vi "cRIO Example FPGA.vi"() -> ()   [LabVIEW 2024]
uses:
  <vilib>/Platform/TimedLoop/XDataNode/timing_clust.ctl
  <vilib>/Platform/TimedLoop/XDataNode/nitl_modes.ctl
  <vilib>/Platform/TimedLoop/XDataNode/wakeup.ctl
  <vilib>/rvi/Emulation/niFpgaSctlEmulationGetInTimedLoop.vi
  <vilib>/rvi/Emulation/niFpgaEmulationReportErrorSimple.vi
  <vilib>/rvi/Emulation/niFpgaGetClockAttributes.vi
  <vilib>/rvi/Emulation/niFpgaCriticalErrorInLSC.vi
  <vilib>/rvi/Emulation/niFpgaProcessEmulError.vi
  <vilib>/rvi/eio/common/nirviEmuTemplateMethod_errors.vi
  <userlib>/_VeriStand FPGA XML Builder/Boolean Array to U64.vi
  <vilib>/NI VeriStand/FPGA/NI VeriStand - Send Packet to Host.vi
  <vilib>/Platform/TimedLoop/XDataNode/XDataNode.xnode
  <vilib>/eio/EIONode/EIONode.xnode
  <userlib>/_VeriStand FPGA XML Builder/FPGA XML.xnode
  <vilib>/Platform/TimedLoop/XDataNode/XDNodeRunTimeDep.lvlib
  <vilib>/NI VeriStand/FPGA/NI_VS FPGA Support.lvlib
panel:
  in  "PulseMeas 0 Timeout":u32=40000
  out "PulseMeas Packet":u64
  in  "Loop Rate (ticks)":u32
  in  "Start":bool
  # "PWM"
  # "Configuration"
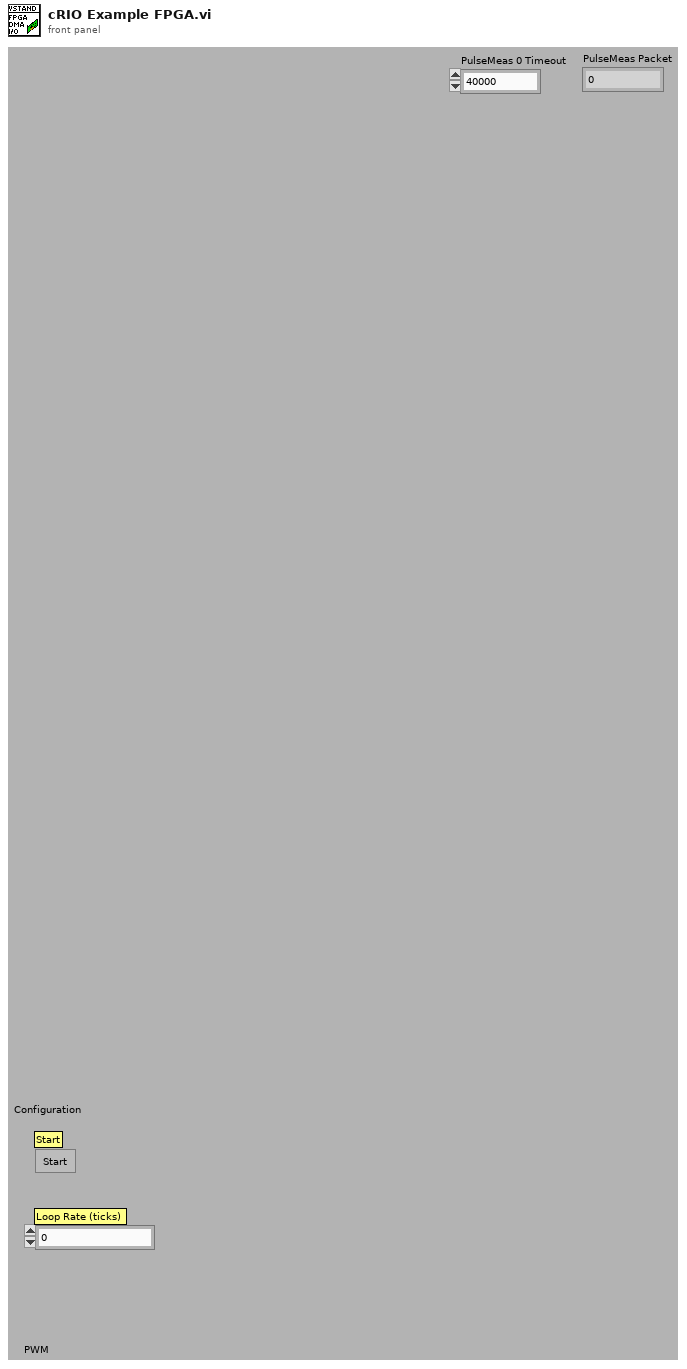
[diagram p1: front panel]
types:
  T1 = typedef "XDNodeRunTimeDep.lvlib/timing_clust.ctl" = cluster{"Expected End [f-1]":u64, "Actual End [f-1]":u64, "Finished Late? [f-1]":bool, "Expected End [i-1]":u64, "Actual End [i-1]":u64, "Finished Late? [i-1]":bool, "Expected Start [i]":u64, "Actual Start [i]":u64, "Expected Start [f]":u64, "Actual Start [f]":u64, "Source Name":string, "Structure Name":string, "Period":i64, "Deadline":i64, "Offset":i64, "Start":i64, "Priority":i32, "Timeout":i32, "Mode":T2, "Wakeup Reason":T3, "Error":errorcluster, "Source Type":string, "Secondary Source Type":string, "Global End Time":u64, "Global Start Time":u64, "Frame Duration":u64, "Iteration Duration":u64, "Assigned CPU":i32, "I/O Scan Engine Mode":u32}
  T2 = typedef "XDNodeRunTimeDep.lvlib/nitl_modes.ctl" = enum32{"No Change", "Process missed periods, maintain original phase", "Discard missed periods, maintain original phase", "Process missed periods, ignore original phase", "Discard missed periods, ignore original phase"}
  T3 = typedef "XDNodeRunTimeDep.lvlib/wakeup.ctl" = enum32{"Normal", "Aborted", "Asynchronous wakeup", "Timing source error", "Timed loop error", "Timeout"}
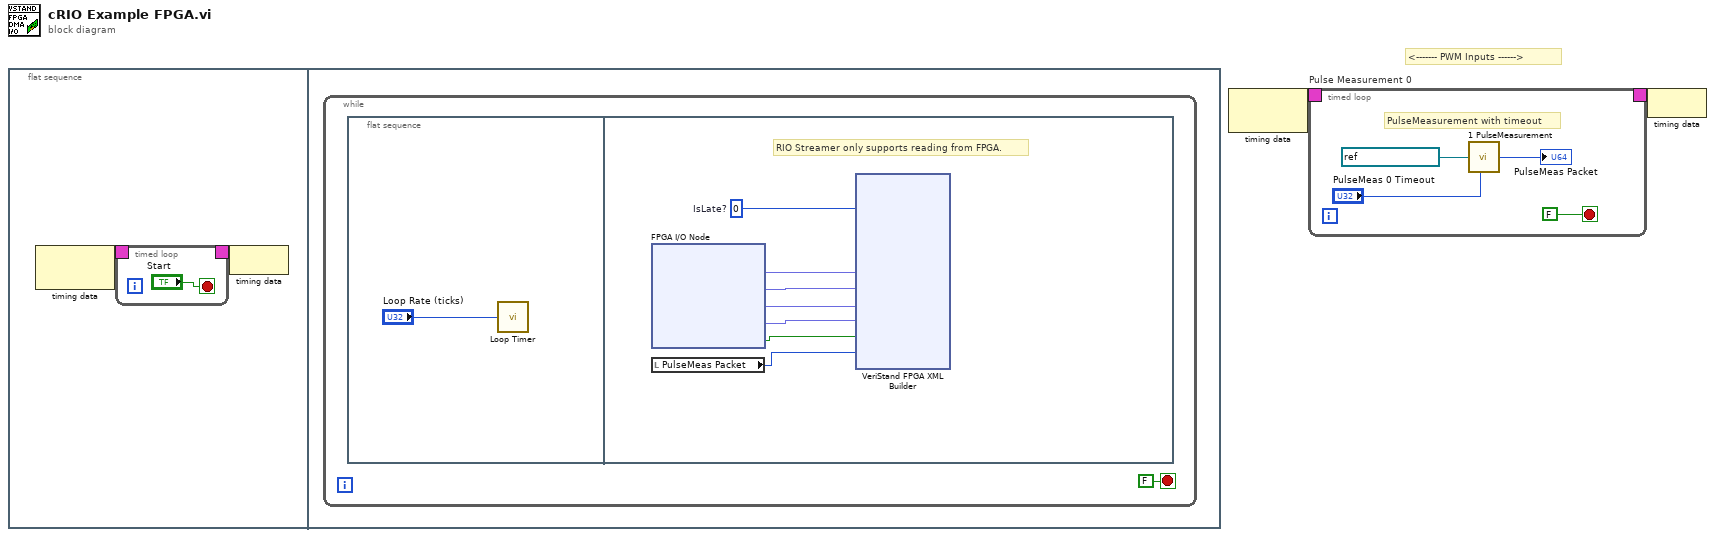
[diagram p0: block diagram]
diagram:
  # "<------- PWM Inputs ------>"
  n1 = flat-sequence {
    frame #0 {
      n2 = node-c288() -> (w4:T1)  [unwired: 1 out]
      n3 = timed-loop {
        timing: w4 -> [_]
        timing-out: [_] -> w3
        stop <- "Start" stop-if-true
      }
      n4 = node-c288(w3) -> ()
    }
    frame #1 {
      n5 = while {
        stop <- FALSE stop-if-true
        n6 = flat-sequence {
          frame #0 {
            n7 = call "Loop Timer"("Count(Ticks)"="Loop Rate (ticks)") -> ()  [unwired: 1 out]
          }
          frame #1 {
            w12 = u64 0  # IsLate?
            # "RIO Streamer only supports reading from FPGA."
            n8 = xnode "FPGA I/O Node"() -> ("NI 9381/AI0"=w18:fxp<+,18,3>, "NI 9381/AI1"=w17:fxp<+,18,3>, "NI 9381/AI2"=w16:fxp<+,18,3>, "NI 9381/AI3"=w15:fxp<+,18,3>, "NI 9381/DIO0"=w14:bool)  [unwired: 5 in, 5 out]
            n9 = local read "PulseMeas Packet"() -> (w13:u64)
            n10 = xnode "VeriStand FPGA XML Builder"("Timing"=w12, "AI0"=w18, "AI1"=w17, "AI2"=w16, "AI3"=w15, "DIO0"=w14, "PWM In 0 (DIO1)"=w13) -> ()
          }
        }
      }
    }
  }
  n11 = node-c288() -> (w2:T1)  [unwired: 1 out]
  n12 = timed-loop "Pulse Measurement 0" {
    timing: w2 -> [_]
    timing-out: [_] -> w1
    stop <- FALSE stop-if-true
    # "PulseMeasurement with timeout"
    n13 = call <userlib>:"1 PulseMeasurement.vi"("PulseMeas Ch"=refnum<k21> "NI 9381/DIO1", "PulseMeas 0 Timeout"="PulseMeas 0 Timeout") -> ("PulseMeas Packet"=→"PulseMeas Packet":u64)  [unwired: 7 in]
  }
  n14 = node-c288(w1) -> ()
